vi "过滤数组元素[CSG].vi"(8 "error in (no error)":errorcluster caption="错误输入（无错误）", 10 "过滤元素":csg[](array[numeric]), 11 "输入数组":csg[](array[numeric])) -> (0 "error out":errorcluster caption="错误输出", 2 "已过滤元素索引":i32[](array[numeric]), 3 "输出数组":csg[](array[numeric]) format="%.2f")   [LabVIEW 2012]
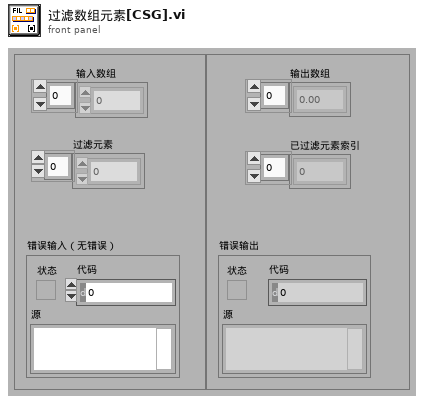
[diagram p1: front panel]
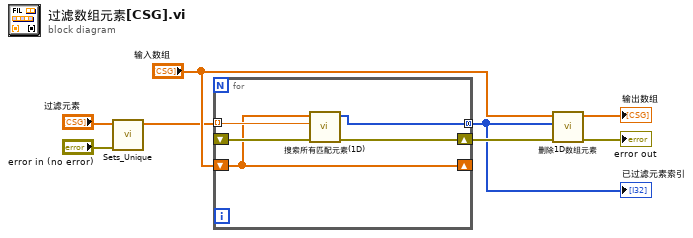
[diagram p0: block diagram]
diagram:
  n1 = call-poly "Sets_Unique.vi"("error in (no error)"="error in (no error)", "输入数组"="过滤元素") -> ("输出数组"=w2:csg[])  [unwired: 7 in, 2 out]
  n2 = for {
    tunnel: w2 -> [w11] mode=indexing
    shift-right: [w10] -> _
    shift-left: "输入数组" -> [w10]
    shift-right: [w12] -> w7
    shift-left: _ -> [w13]
    tunnel: [w9] -> w1 mode=concatenating
    n3 = call-poly "搜索所有匹配元素(1D).vi"("error in (no error)"=w13, "元素"=w11, "数组"=w10) -> ("error out"=w12:errorcluster, "匹配元素索引"=w9:i32[])  [unwired: 6 in, 1 out]
  }
  "已过滤元素索引" <- w1
  n4 = call-poly "删除1D数组元素.vi"("error in (no error)"=w7, "索引"=w1, "输入数组"="输入数组") -> ("error out"=→"error out":errorcluster, "剩余元素"=→"输出数组":csg[])  [unwired: 6 in, 1 out]
